vi "428_DATA (SubVI).vi"(1 "read buffer":string) -> (0 "trimmed string":string)   [LabVIEW 2016]
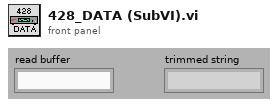
[diagram p1: front panel]
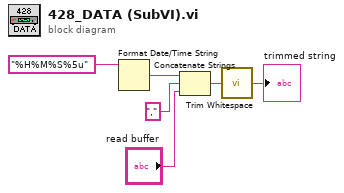
[diagram p0: block diagram]
diagram:
  n1 = Format Date/Time String(time format string (%c)="%H%M%S%5u") -> (date/time string=w6:string)  [unwired: 2 in]
  n2 = Concatenate Strings(w6, ",", "read buffer") -> (w2:string)
  n3 = call <vilib>:"Trim Whitespace.vi"("string"=w2) -> ("trimmed string"=→"trimmed string":string)  [unwired: 1 in]
